vi "get_am_presence.vi"(6 "timeout (25000ms)":i32=25000, 8 "error in (no error)":errorcluster, 11 "daemon reference in":refnum<k5>) -> (0 "error out":errorcluster, 1 "presence?":bool, 2 "response":string, 3 "daemon reference out":refnum<k5>, 5 "command out":string="random")   [LabVIEW 2017]
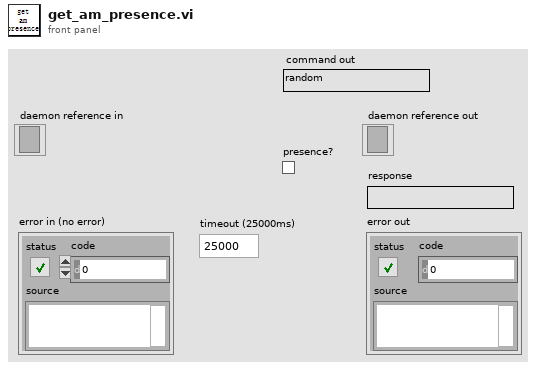
[diagram p1: front panel]
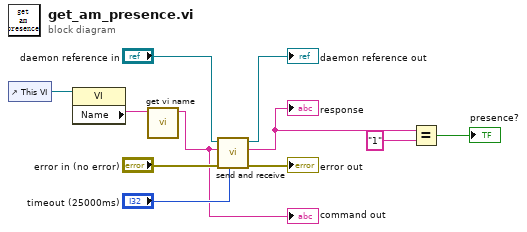
[diagram p0: block diagram]
diagram:
  n1 = control-ref of="This VI"() -> (w6:refnum<vi>)
  n2 = property class="VI"(reference=w6) -> ("Name"=w5:string)  [unwired: 1 in, 2 out]
  n3 = call "get vi name.vi"("library.lvlib:name.vi"=w5) -> ("vi name"=w4:string)  [unwired: 10 in]
  "command out" <- w4
  n4 = call "send and receive.vi"("timeout (25000ms)"="timeout (25000ms)", "error in (no error)"="error in (no error)", "command"=w4, "daemon reference in"="daemon reference in") -> ("error out"=→"error out":errorcluster, "response"=w3:string, "daemon reference out"=→"daemon reference out":refnum<k5>)  [unwired: 5 in]
  "response" <- w3
  n5 = Equal?(x=w3, y="1") -> (x = y?=→"presence?":bool)
